vi "FGV GaseRing aendern.vi"() -> ()   [LabVIEW 2015, in "Linearisierung v2.lvlib" / "Gasteiler.lvlib" / "HovaCal.lvlib"]
uses:
  HovaCal.lvlib
panel:
  out "Gase 2":cluster{string, i32}[](array[cluster])
  in  "Gase":cluster{string, i32}[][](array[cluster])
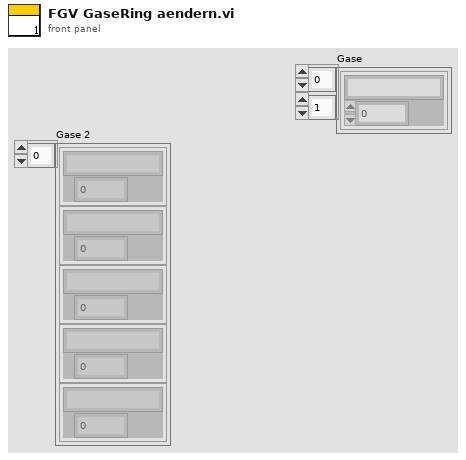
[diagram p1: front panel]
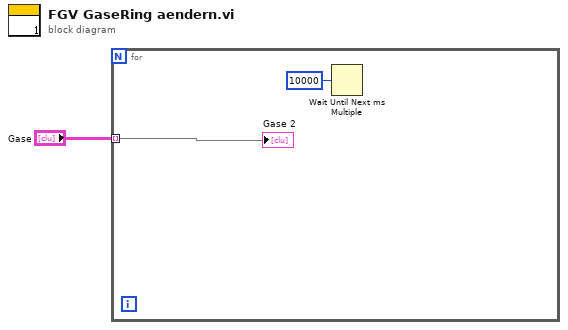
[diagram p0: block diagram]
diagram:
  n1 = for {
    tunnel: "Gase" -> [w3] mode=indexing
    n2 = Wait Until Next ms Multiple(millisecond multiple=u32 10000 ("ms")) -> ()  [unwired: 1 out]
    "Gase 2" <- w3
  }
